vi "FullArrayConvolve.vi"(4 "rings":dbl[](array[numeric]), 6 "DR Inputs":T1 {"Tansducer" items=["F2 40 MHz", "F3 20 MHz"]}, 7 "Recip Processing":u16[][](array[ring])=[[1, 1, 1, 1, 1], [1, 1, 1, 1, 1], [1, 1, 1, 1, 1], [1, 1, 1, 1, 1], [1, 1, 1, 1, 1]] items=["0", "1", "2"], 8 "Variables":T2={"Number of rings"=1, "sound spd (cm/s)"=150000, "z span (cm)"=4.0, "z steps"=20, "y spacing (cm)"=0.01, "y steps"=50, "time step (s)"=1e-08, "z"=0.0, "y"=0.0, "ref delay"=0.0, "freq (MHz)"=4.71, "cycles"=300} {"freq (MHz)" format="%.2f"; "z span (cm)" format="%.2f"; "y" format="%.2f"; "ref delay" format="%.2f"; "y spacing (cm)" format="%.2f"; "z" format="%.2f"; "time step (s)" format="%.2e"}, 9 "delay pts":i32[][](array[numeric]), 10 "h(r,t)":dbl[][][](array[numeric]) format="%.2f", 11 "Rings":T3(array[cluster]) {"focus delay abs (s)" format="%.2e"; "Waveform" format="%.2f"; "Annular rings"."a" format="%.2f"; "Annular rings"."Radius" format="%.2f"}) -> (2 "data out":dbl[][](array[numeric]))   [LabVIEW 2022 SP3]
panel:
  # "If true it used a fixed transmit delay at geometric focus.\nNeed to make diagram change to transmit focus elsewhere."
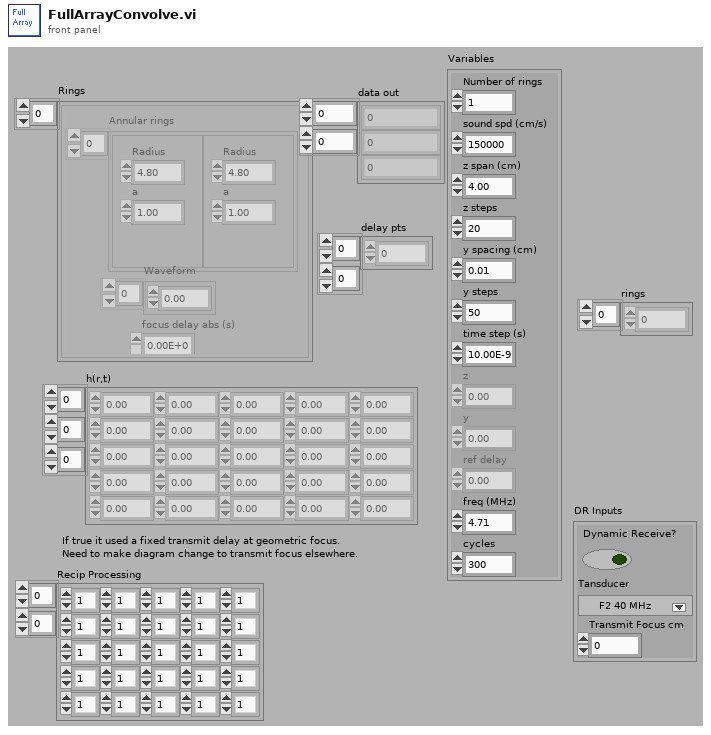
[diagram p1: front panel]
types:
  T1 = cluster{"Dynamic Receive?":bool, "Tansducer":u16, "Transmit Focus cm":dbl}
  T2 = cluster{"Number of rings":i32, "sound spd (cm/s)":i32, "z span (cm)":dbl, "z steps":i32, "y spacing (cm)":dbl, "y steps":i32, "time step (s)":sgl, "z":dbl, "y":dbl, "ref delay":dbl, "freq (MHz)":dbl, "cycles":i32}
  T3 = cluster{"Annular rings":cluster{"Radius":dbl, "a":dbl}[], "Waveform":dbl[], "focus delay abs (s)":dbl}[]
  T4 = cluster{"Annular rings":cluster{"Radius":dbl, "a":dbl}[], "Waveform":dbl[], "focus delay abs (s)":dbl}
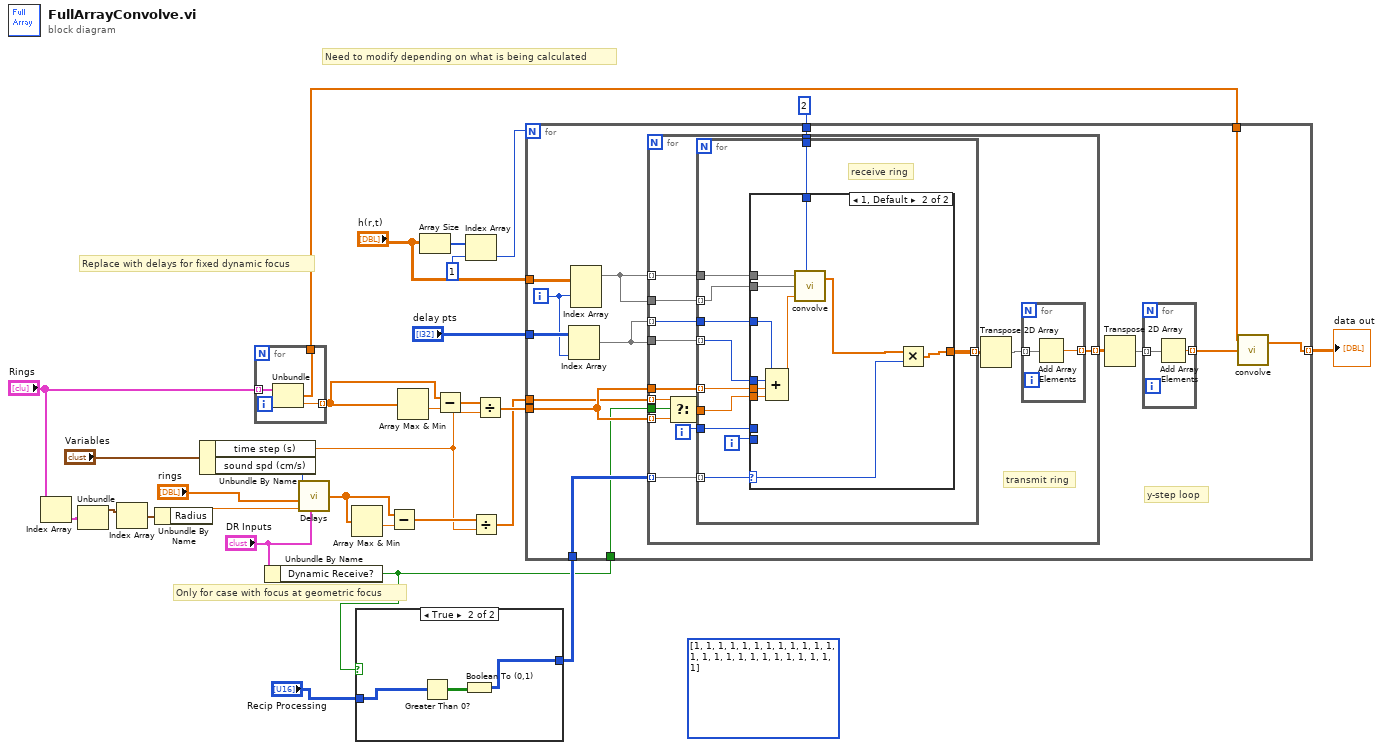
[diagram p0: block diagram]
diagram:
  (unwired) u16[][] [[1, 1, 1, 1, 1], [1, 1, 1, 1, 1], [1, 1, 1, 1, 1], [1, 1, 1, 1, 1], [1, 1, 1, 1, 1]] items=["0", "1", "2"] ("Recip Processing")
  # "Only for case with focus at geometric focus"
  # "Replace with delays for fixed dynamic focus"
  # "Need to modify depending on what is being calculated"
  n1 = Index Array(array="Rings") -> (element=w6:T4)  [unwired: 1 in]
  n2 = Unbundle(w6) -> ("Annular rings"=w5:cluster{"Radius":dbl, "a":dbl}[])  [unwired: 2 out]
  n3 = Index Array(array=w5) -> (element=w4:cluster{"Radius":dbl, "a":dbl})  [unwired: 1 in]
  n4 = Unbundle By Name(w4) -> ("Radius"=w3:dbl)
  n5 = Unbundle By Name("Variables") -> ("time step (s)"=w13:sgl, "sound spd (cm/s)"=w11:i32)
  n6 = for {
    tunnel: "Rings" -> [w32] mode=indexing
    tunnel: [w31] -> w27 mode=indexing
    tunnel: [w30] -> w14
    n7 = Unbundle(w32) -> ("Waveform"=w30:dbl[], "focus delay abs (s)"=w31:dbl)  [unwired: 1 out]
  }
  n8 = Unbundle By Name("DR Inputs") -> ("Dynamic Receive?"=w9:bool)
  n9 = call "Delays.vi"("sound spd (cm/s)"=w11, "rings"="rings", "radius"=w3, "DR Inputs"="DR Inputs") -> ("delays"=w12:dbl[])  [unwired: 1 out]
  n10 = Array Max & Min(array=w12) -> (min value=w17:dbl)  [unwired: 3 out]
  n11 = case shown="True" w9 {
    tunnel: [w33 w34] -> w18
    tunnel: "Recip Processing" -> [w33 w35]
    frame False {
    }
    frame True {
      n12 = Greater Than 0?(x=w35) -> (x > 0?=w36:bool[][])
      n13 = Boolean To (0,1)(Boolean=w36) -> (0, 1=w34:i16[][])
    }
  }
  n14 = Subtract(x=w12, y=w17) -> (x-y=w16:dbl[])
  n15 = Array Max & Min(array=w27) -> (min value=w29:dbl)  [unwired: 3 out]
  n16 = Array Size(array="h(r,t)") -> (size(s)=w26:i32[])
  n17 = Subtract(x=w27, y=w29) -> (x-y=w28:dbl[])
  n18 = Index Array(array=w26, index=1) -> (element=w24:i32)
  n19 = Divide(x=w16, y=w13) -> (x/y=w15:dbl[])
  n20 = Divide(x=w28, y=w13) -> (x/y=w22:dbl[])
  n21 = for {
    N: w24 -> [_]
    tunnel: "h(r,t)" -> [w51]
    tunnel: "delay pts" -> [w49]
    tunnel: w22 -> [w39]
    tunnel: w14 -> [w40]
    tunnel: [w41] -> w20 mode=indexing
    tunnel: 2 -> [w44]
    tunnel: w18 -> [w43]
    tunnel: w15 -> [w38]
    tunnel: w9 -> [w37]
    i -> [w47]
    # "y-step loop"
    n22 = Index Array(array=w49, index (col)=w47) -> (element=w48:i32[])  [unwired: 1 in]
    n23 = Index Array(array=w51, index (dim 1)=w47) -> (element=w50:dbl[][])  [unwired: 2 in]
    n24 = for {
      tunnel: w50 -> [w68]
      tunnel: w50 -> [w65] mode=indexing
      tunnel: w48 -> [w67]
      tunnel: w48 -> [w66] mode=indexing
      tunnel: w39 -> [w56] mode=indexing
      tunnel: w39 -> [w64]
      tunnel: [w62] -> w45 mode=indexing
      tunnel: w44 -> [w60]
      tunnel: w43 -> [w59] mode=indexing
      tunnel: w38 -> [w55] mode=indexing
      tunnel: w37 -> [w54]
      i -> [w58]
      # "transmit ring"
      n25 = Select(t=w55, s=w54, f=w56) -> (s? t:f=w57:dbl)
      n26 = for {
        tunnel: w65 -> [w80]
        tunnel: w68 -> [w79] mode=indexing
        tunnel: w67 -> [w76] mode=indexing
        tunnel: w66 -> [w77]
        tunnel: w64 -> [w81] mode=indexing
        tunnel: [w72] -> w63 mode=indexing
        tunnel: w57 -> [w78]
        tunnel: w60 -> [w75]
        tunnel: w59 -> [w71] mode=indexing
        tunnel: w58 -> [w74]
        i -> [w73]
        # "receive ring"
        n27 = case shown="1, Default" w71 {
          selector: w71 -> [_ w82]
          tunnel: w81 -> [_ w92]
          tunnel: w80 -> [_ w91]
          tunnel: w79 -> [_ w90]
          tunnel: w78 -> [_ w89]
          tunnel: w77 -> [_ w88]
          tunnel: w76 -> [_ w87]
          tunnel: w75 -> [_ w86]
          tunnel: w74 -> [_ _]
          tunnel: w73 -> [_ _]
          tunnel: [_ w84] -> w72
          frame 0 {
          }
          frame 1, Default {
            n28 = Compound Arithmetic op=ADD(w88, w87, w92, w89) -> (w85:dbl)
            n29 = call "convolve.vi"("X"=w91, "Calc"=w86, "Y"=w90, "delay pts"=w85) -> ("X*Y"=w83:dbl[])  [unwired: 2 out]
            n30 = Multiply(x=w83, y=w82) -> (x*y=w84:dbl[])
          }
        }
      }
      n31 = Transpose 2D Array(2D array=w63) -> (transposed array=w61:dbl[][])
      n32 = for {
        tunnel: w61 -> [w70] mode=indexing
        tunnel: [w69] -> w62 mode=indexing
        n33 = Add Array Elements(numeric array=w70) -> (sum=w69:dbl)
      }
    }
    n34 = Transpose 2D Array(2D array=w45) -> (transposed array=w46:dbl[][])
    n35 = for {
      tunnel: w46 -> [w53] mode=indexing
      tunnel: [w52] -> w42 mode=indexing
      n36 = Add Array Elements(numeric array=w53) -> (sum=w52:dbl)
    }
    n37 = call "convolve.vi"("X"=w40, "Y"=w42) -> ("X*Y"=w41:dbl[])  [unwired: 2 in, 2 out]
  }
  "data out" <- w20
